vi "AE DataProcessControl.vi"(7 "Action":T1, 8 "error in (no error)":errorcluster, 9 "Cursor Mode In":bool, 10 "Data Path In":path) -> (0 "error out":errorcluster, 1 "Cursor Mode Out":bool, 2 "Data Path Out":path)   [LabVIEW 2013, in "main.lvlib"]
uses:
  main.lvlib
  Controls/Enum Process Data.ctl
  Controls/Cluster Process Data.ctl
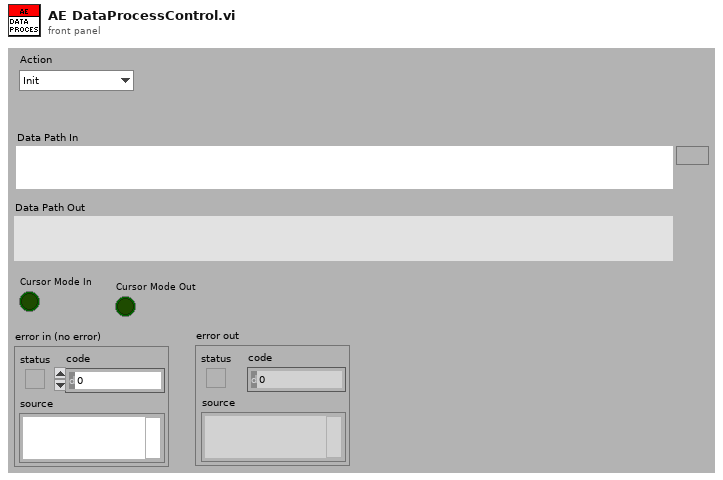
[diagram p1: front panel]
types:
  T1 = typedef "main.lvlib/Enum Process Data.ctl" = enum16{"Init", "Set Cursor Mode", "Set Data Path", "Get All"}
  T2 = typedef "main.lvlib/Cluster Process Data.ctl" = cluster{"DataFile":path, "Cursor Mode":bool}
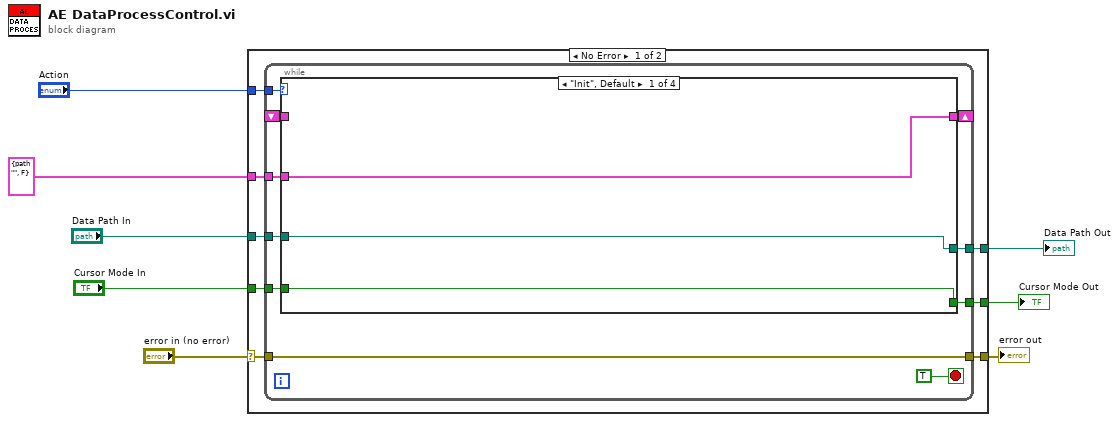
[diagram p0: block diagram]
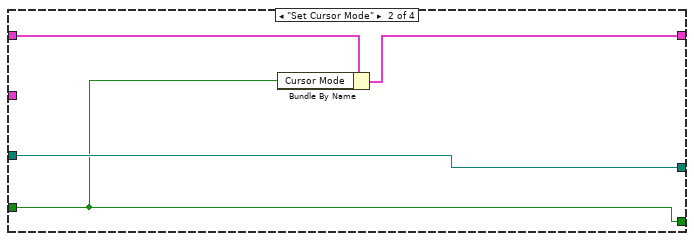
[diagram p2: hidden frame]
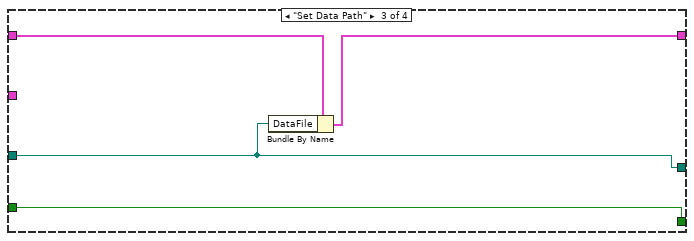
[diagram p3: hidden frame]
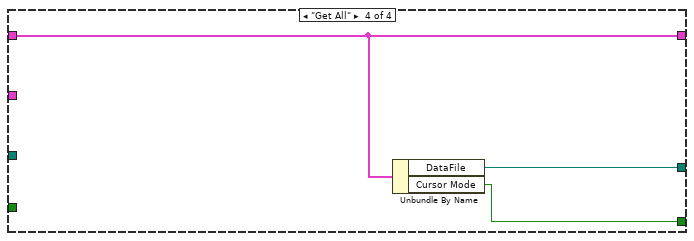
[diagram p4: hidden frame]
diagram:
  n1 = case shown="No Error" "error in (no error)" {
    selector: "error in (no error)" -> [w11 w43]
    tunnel: T2 {"DataFile"=path "", "Cursor Mode"=FALSE} ("Cluster") -> [w16 _]
    tunnel: [w15 w42] -> w7
    tunnel: "Data Path In" -> [w14 w42]
    tunnel: "Action" -> [w13 _]
    tunnel: [w12 w43] -> w4
    tunnel: "Cursor Mode In" -> [w10 w41]
    tunnel: [w9 w41] -> w1
    frame No Error {
      n2 = while {
        shift-right: [w25] -> _
        shift-left: _ -> [w23]
        tunnel: w13 -> [w26]
        tunnel: w16 -> [w24]
        tunnel: [w22] -> w15
        tunnel: w14 -> [w21]
        tunnel: [w20] -> w12
        tunnel: w11 -> [w20]
        tunnel: w10 -> [w18]
        tunnel: [w17] -> w9
        stop <- TRUE stop-if-true
        n3 = case shown="\"Init\", Default" w26 {
          tunnel: [w27 w32 w36 w40] -> w25
          tunnel: w24 -> [w27 _ _ _]
          tunnel: w23 -> [_ w33 w37 w40]
          tunnel: [w29 w31 w35 w39] -> w22
          tunnel: w21 -> [w29 w31 w35 _]
          tunnel: w18 -> [w28 w30 w34 _]
          tunnel: [w28 w30 w34 w38] -> w17
          frame "Init", Default {
          }
          frame "Set Cursor Mode" {
            n4 = Bundle By Name(cluster=w33, "Cursor Mode"=w30) -> (w32:T2)
          }
          frame "Set Data Path" {
            n5 = Bundle By Name(cluster=w37, "DataFile"=w35) -> (w36:T2)
          }
          frame "Get All" {
            n6 = Unbundle By Name(w40) -> ("DataFile"=w39:path, "Cursor Mode"=w38:bool)
          }
        }
      }
    }
    frame Error {
    }
  }
  "Data Path Out" <- w7
  "error out" <- w4
  "Cursor Mode Out" <- w1
